vi "Convert PID Gains (PID).vi"(0 "proportional":sgl, 1 "gains pattern (Parallel)":T4=1 items=["Academic", "Parallel", "Series"], 2 "filter coefficient (NaN)":sgl=nan, 3 "filter coefficient unit (Alpha)":T1 items=["Alpha", "N", "Cutoff Frequency", "Time Constant"], 5 "integral":sgl, 7 "derivative":sgl, 9 "sampling time":sgl min=0, 11 "error in (no error)":errorcluster, 12 "proportional unit (Gain (K))":T3 items=["Gain (K)", "Band (PB)"], 13 "integral unit (Hz)":T2 items=["Hz", "s", "min"], 14 "derivative unit (s)":T2=1 items=["Hz", "s", "min"]) -> (4 "gains":T5 {"proportional gain" step=0.125}, 15 "error out":errorcluster)   [LabVIEW 2020]
doc: "Converts PID gains in the Academic, Parallel, or Series form to the normalized Parallel form that the PID VI expects."
uses:
  <vilib>/rvi/Analysis/control/PID/Typedef/niFpgaPID_PIDGains.ctl
  <vilib>/rvi/Analysis/host/Private/PID Gains Pattern.ctl
  <vilib>/rvi/Analysis/host/Private/PID Proportional Unit.ctl
  <vilib>/rvi/Analysis/host/Private/PID Integral Derivative Unit.ctl
  <vilib>/rvi/Analysis/host/Private/PID Filter Coefficient Unit.ctl
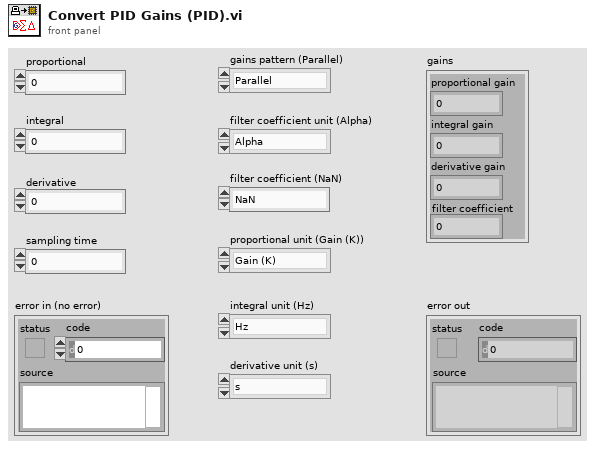
[diagram p1: front panel]
types:
  T1 = typedef "PID Filter Coefficient Unit.ctl" = u8
  T2 = typedef "PID Integral Derivative Unit.ctl" = u8
  T3 = typedef "PID Proportional Unit.ctl" = u8
  T4 = typedef "PID Gains Pattern.ctl" = u8
  T5 = typedef "niFpgaPID_PIDGains.ctl" = cluster{"proportional gain":sgl, "integral gain":sgl, "derivative gain":sgl, "filter coefficient":sgl}
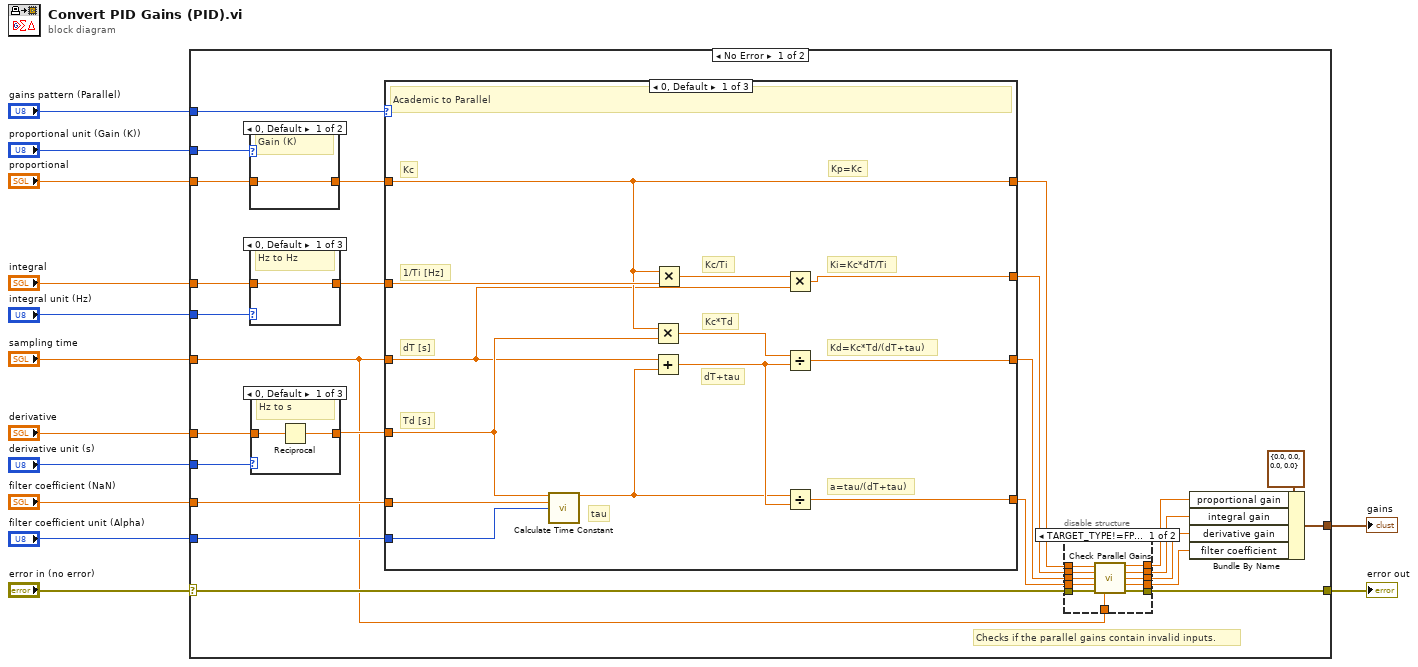
[diagram p0: block diagram]
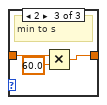
[diagram p4: hidden frame]
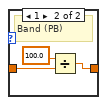
[diagram p5: hidden frame]
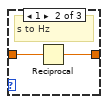
[diagram p6: hidden frame]
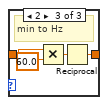
[diagram p7: hidden frame]
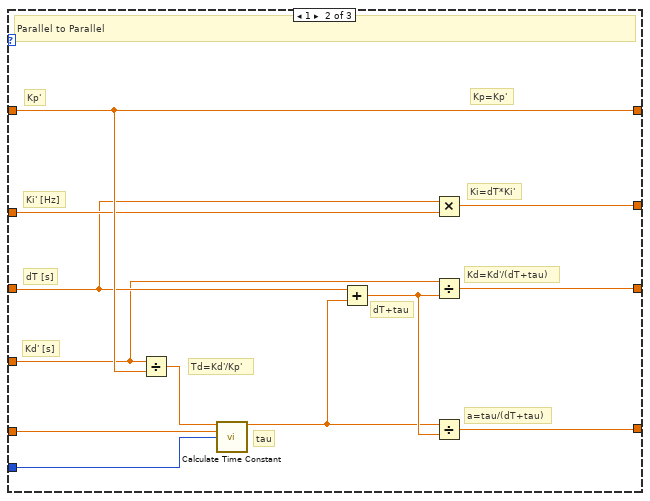
[diagram p8: hidden frame]
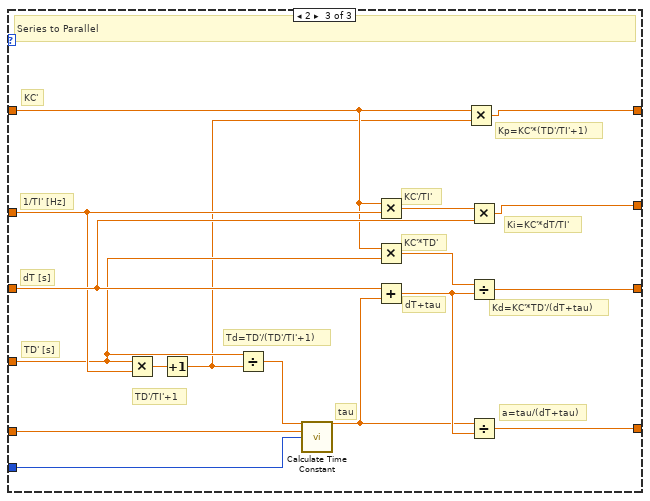
[diagram p9: hidden frame]
diagram:
  n1 = case shown="No Error" "error in (no error)" {
    selector: "error in (no error)" -> [w34 w114]
    tunnel: "gains pattern (Parallel)" -> [w38 _]
    tunnel: "proportional" -> [w26 _]
    tunnel: "integral" -> [w28 _]
    tunnel: "filter coefficient (NaN)" -> [w37 _]
    tunnel: "sampling time" -> [w14 _]
    tunnel: "filter coefficient unit (Alpha)" -> [w36 _]
    tunnel: [w35 w114] -> w11
    tunnel: "proportional unit (Gain (K))" -> [w25 _]
    tunnel: "integral unit (Hz)" -> [w24 _]
    tunnel: "derivative" -> [w22 _]
    tunnel: "derivative unit (s)" -> [w21 _]
    tunnel: [w20 _] -> w6
    frame No Error {
      # "Checks if the parallel gains contain invalid inputs."
      n2 = case shown="0, Default" w25 {
        tunnel: w26 -> [w61 w62]
        tunnel: [w61 w64] -> w27
        frame 0, Default {
          # "Gain (K)"
        }
        frame 1 {
          # "Band (PB)"
          n3 = Divide(x=sgl 100.0, y=w62) -> (x/y=w64:sgl)
        }
      }
      n4 = case shown="0, Default" w24 {
        tunnel: w28 -> [w65 w66 w70]
        tunnel: [w65 w67 w68] -> w29
        frame 0, Default {
          # "Hz to Hz"
        }
        frame 1 {
          # "s to Hz"
          n5 = Reciprocal(x=w66) -> (1/x=w67:sgl)
        }
        frame 2 {
          # "min to Hz"
          n6 = Multiply(x=w70, y=sgl 60.0) -> (x*y=w71:sgl)
          n7 = Reciprocal(x=w71) -> (1/x=w68:sgl)
        }
      }
      n8 = case shown="0, Default" w21 {
        tunnel: w22 -> [w56 w57 w58]
        tunnel: [w55 w57 w59] -> w23
        frame 0, Default {
          # "Hz to s"
          n9 = Reciprocal(x=w56) -> (1/x=w55:sgl)
        }
        frame 1 {
          # "s to s"
        }
        frame 2 {
          # "min to s"
          n10 = Multiply(x=w58, y=sgl 60.0) -> (x*y=w59:sgl)
        }
      }
      n11 = case shown="0, Default" w38 {
        tunnel: w27 -> [w75 w95 w98]
        tunnel: w29 -> [w83 w94 w101]
        tunnel: w23 -> [w77 w89 w99]
        tunnel: w37 -> [w78 w87 w107]
        tunnel: w14 -> [w72 w93 w110]
        tunnel: w36 -> [w79 w86 w108]
        tunnel: [w84 w96 w111] -> w30
        tunnel: [w75 w95 w109] -> w33
        tunnel: [w73 w92 w113] -> w32
        tunnel: [w80 w91 w112] -> w31
        frame 0, Default {
          # "Kp=Kc"
          # "Kd=Kc*Td/(dT+tau)"
          # "Kc*Td"
          # "Ki=Kc*dT/Ti"
          # "Kc/Ti"
          # "dT+tau"
          # "a=tau/(dT+tau)"
          # "dT [s]"
          # "tau"
          # "Kc"
          # "1/Ti [Hz]"
          # "Td [s]"
          # "Academic to Parallel"
          n12 = call <vilib>:"Calculate Time Constant.vi"("derivative time"=w77, "filter coefficient (NaN)"=w78, "filter coefficient unit (Alpha)"=w79) -> ("time constant"=w76:sgl)  [unwired: 12 in]
          n13 = Multiply(x=w75, y=w77) -> (x*y=w82:sgl)
          n14 = Add(x=w72, y=w76) -> (x+y=w81:sgl)
          n15 = Multiply(x=w75, y=w83) -> (x*y=w74:sgl)
          n16 = Multiply(x=w74, y=w72) -> (x*y=w73:sgl)
          n17 = Divide(x=w82, y=w81) -> (x/y=w80:sgl)
          n18 = Divide(x=w76, y=w81) -> (x/y=w84:sgl)
        }
        frame 1 {
          # "Kp=Kp'"
          # "dT [s]"
          # "Ki=dT*Ki'"
          # "Kd=Kd'/(dT+tau)"
          # "dT+tau"
          # "tau"
          # "a=tau/(dT+tau)"
          # "Td=Kd'/Kp'"
          # "Kp'"
          # "Ki' [Hz]"
          # "Kd' [s]"
          # "Parallel to Parallel"
          n19 = Divide(x=w89, y=w95) -> (x/y=w88:sgl)
          n20 = call <vilib>:"Calculate Time Constant.vi"("derivative time"=w88, "filter coefficient (NaN)"=w87, "filter coefficient unit (Alpha)"=w86) -> ("time constant"=w85:sgl)  [unwired: 12 in]
          n21 = Add(x=w93, y=w85) -> (x+y=w90:sgl)
          n22 = Multiply(x=w93, y=w94) -> (x*y=w92:sgl)
          n23 = Divide(x=w89, y=w90) -> (x/y=w91:sgl)
          n24 = Divide(x=w85, y=w90) -> (x/y=w96:sgl)
        }
        frame 2 {
          # "TD'/TI'+1"
          # "Kd=KC'*TD'/(dT+tau)"
          # "KC'*TD'"
          # "Ki=KC'*dT/TI'"
          # "KC'/TI'"
          # "Kp=KC'*(TD'/TI'+1)"
          # "dT+tau"
          # "a=tau/(dT+tau)"
          # "tau"
          # "Td=TD'/(TD'/TI'+1)"
          # "dT [s]"
          # "TD' [s]"
          # "1/TI' [Hz]"
          # "KC'"
          # "Series to Parallel"
          n25 = Multiply(x=w99, y=w101) -> (x*y=w100:sgl)
          n26 = Increment(x=w100) -> (x+1=w97:sgl)
          n27 = Divide(x=w99, y=w97) -> (x/y=w103:sgl)
          n28 = call <vilib>:"Calculate Time Constant.vi"("derivative time"=w103, "filter coefficient (NaN)"=w107, "filter coefficient unit (Alpha)"=w108) -> ("time constant"=w102:sgl)  [unwired: 12 in]
          n29 = Multiply(x=w98, y=w101) -> (x*y=w106:sgl)
          n30 = Multiply(x=w98, y=w99) -> (x*y=w105:sgl)
          n31 = Add(x=w110, y=w102) -> (x+y=w104:sgl)
          n32 = Multiply(x=w98, y=w97) -> (x*y=w109:sgl)
          n33 = Multiply(x=w106, y=w110) -> (x*y=w113:sgl)
          n34 = Divide(x=w105, y=w104) -> (x/y=w112:sgl)
          n35 = Divide(x=w102, y=w104) -> (x/y=w111:sgl)
        }
      }
      n36 = disable-structure shown="TARGET_TYPE!=FPGA, Default" {
        disable-tunnel: [w49 w54] -> w35
        disable-tunnel: w34 -> [w48 w54]
        disable-tunnel: w33 -> [w47 w53]
        disable-tunnel: w32 -> [w46 w52]
        disable-tunnel: w31 -> [w45 w51]
        disable-tunnel: w30 -> [w44 w50]
        disable-tunnel: [w43 w53] -> w18
        disable-tunnel: [w42 w52] -> w17
        disable-tunnel: [w41 w51] -> w16
        disable-tunnel: [w40 w50] -> w15
        disable-tunnel: w14 -> [w39 _]
        frame condition #0 (active) {
          n37 = call <vilib>:"Check Parallel Gains.vi"("proportional gain in"=w47, "integral gain in (0)"=w46, "derivative gain in (0)"=w45, "filter coefficient in (0)"=w44, "error in (no error)"=w48, "sampling time"=w39) -> ("proportional gain out"=w43:sgl, "integral gain out"=w42:sgl, "derivative gain out"=w41:sgl, "filter coefficient out"=w40:sgl, "error out"=w49:errorcluster)  [unwired: 5 in]
        }
        frame condition #1 {
        }
      }
      n38 = Bundle By Name(cluster=T5 {"proportional gain"=0.0, "integral gain"=0.0, "derivative gain"=0.0, "filter coefficient"=0.0} ("gains"), "proportional gain"=w18, "integral gain"=w17, "derivative gain"=w16, "filter coefficient"=w15) -> (w20:T5)
    }
    frame Error {
    }
  }
  "error out" <- w11
  "gains" <- w6
